vi "Initialize Measurement Actor Core.vi"(5 "Title Ref":refnum<vi>, 7 "Wvfm Graph Ref":refnum<vi>, 8 "error in (no error)":errorcluster, 11 "Measurement in":refnum<class "Function.lvclass">) -> (0 "error out":errorcluster, 1 "event out":refnum<user-event>, 2 "notifier out":refnum<notifier>, 3 "Measurement out":refnum<class "Function.lvclass">)   [LabVIEW 2016, in "Function Actor.lvlib" / "Function.lvclass"]
uses:
  <userlib>/Common Components/Function Actor/Function.lvclass
  C:/Program Files (x86)/National Instruments/LabVIEW 2016/vi.lib/ActorFramework/Actor/Actor.lvclass
  <userlib>/Common Components/Function Actor/Function.lvclass/Function.ctl
  <vilib>/ActorFramework/Actor/Actor.lvclass/Actor.ctl
  <vilib>/ActorFramework/Message Enqueuer/Message Enqueuer.lvclass/Message Enqueuer.ctl
  <vilib>/ActorFramework/Message Enqueuer/Enqueue.vi
  <vilib>/ActorFramework/Message Enqueuer/Init from Existing Queue.vi
  <userlib>/Common Components/Function Actor/Messages/Configure Msg/Configure Msg.lvclass
  C:/Program Files (x86)/National Instruments/LabVIEW 2016/vi.lib/ActorFramework/Message/Message.lvclass
  <vilib>/ActorFramework/Message Priority Queue/Priority Enqueue.vi
  <vilib>/ActorFramework/Message Enqueuer/Message Enqueuer.lvclass
  <vilib>/ActorFramework/Actor/Actor.lvclass
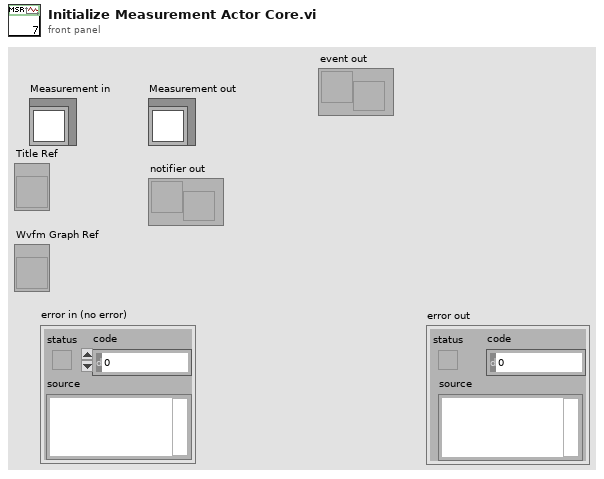
[diagram p1: front panel]
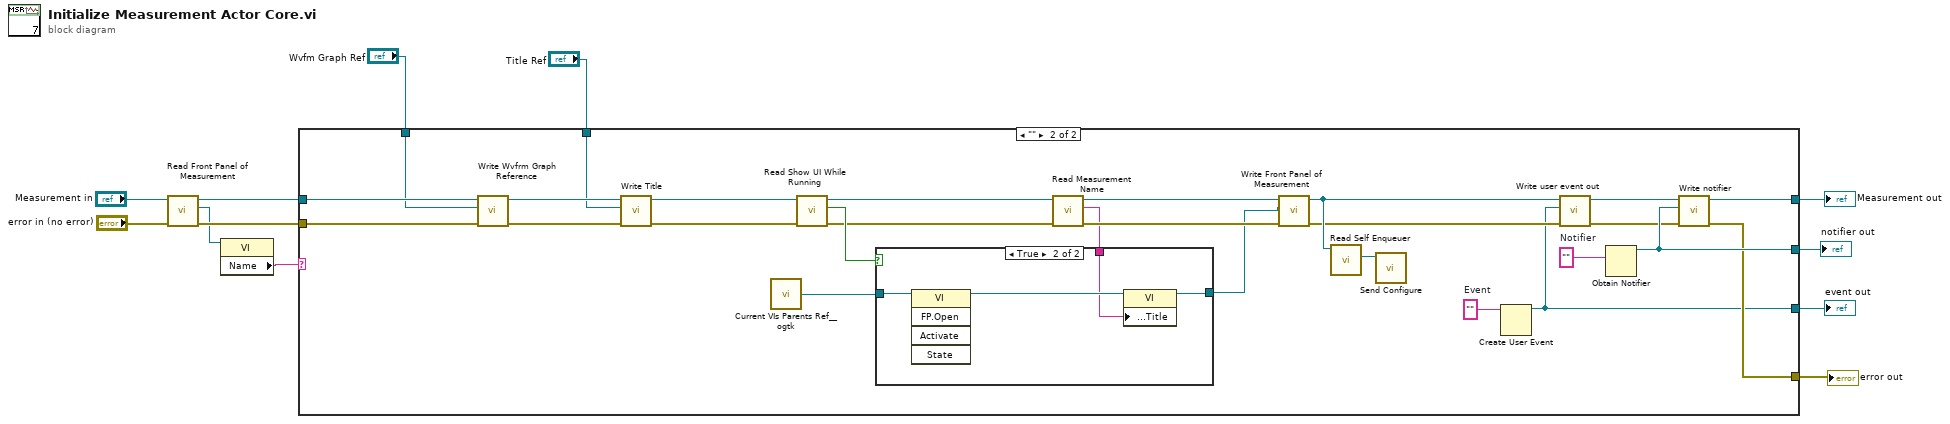
[diagram p0: block diagram]
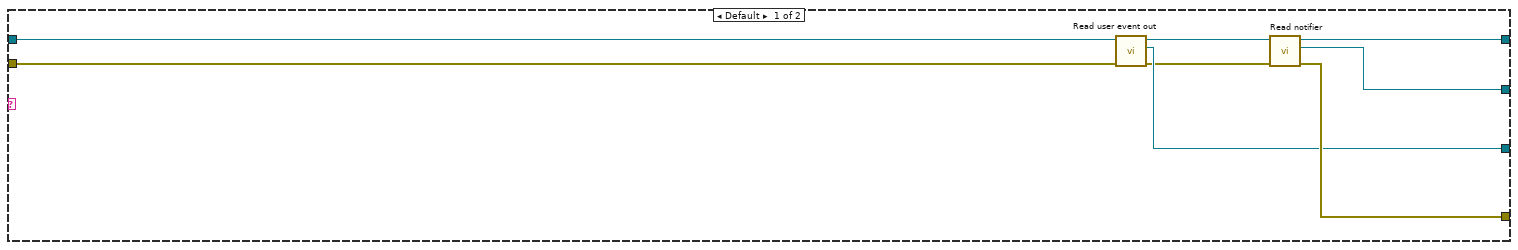
[diagram p2: hidden frame]
diagram:
  n1 = call <userlib>:"Read Front Panel of Measurement.vi"("error in (no error)"="error in (no error)", "Measurement in"="Measurement in") -> ("error out"=w9:errorcluster, "Front Panel of Measurement"=w8:refnum<vi>, "Measurement out"=w10:refnum<class "Function.lvclass">)  [unwired: 7 in]
  n2 = property class="VI"(reference=w8) -> ("Name"=w7:string)  [unwired: 1 in, 2 out]
  n3 = case shown="\"\"" w7 {
    tunnel: [w20 w46] -> w5
    tunnel: w10 -> [w17 w28]
    tunnel: w9 -> [w14 w27]
    tunnel: [w19 w45] -> w6
    tunnel: [w18 w44] -> w4
    tunnel: [w15 w29] -> w3
    tunnel: "Title Ref" -> [_ w22]
    tunnel: "Wvfm Graph Ref" -> [_ w21]
    frame Default {
      n4 = call <userlib>:"Read user event out.vi"("error in (no error)"=w14, "Measurement in"=w17) -> ("error out"=w13:errorcluster, "user event out"=w15:refnum<user-event>, "Measurement out"=w16:refnum<class "Function.lvclass">)  [unwired: 7 in]
      n5 = call <userlib>:"Read notifier.vi"("error in (no error)"=w13, "Measurement in"=w16) -> ("error out"=w18:errorcluster, "notifier"=w19:refnum<notifier>, "Measurement out"=w20:refnum<class "Function.lvclass">)  [unwired: 7 in]
    }
    frame "" {
      w34 = ""  # Event
      w47 = ""  # Notifier
      n6 = call <userlib>:"Write Wvfrm Graph Reference.vi"("error in (no error)"=w27, "General Measurement UI"=w21, "Measurement in"=w28) -> ("error out"=w26:errorcluster, "Measurement out"=w25:refnum<class "Function.lvclass">)  [unwired: 7 in]
      n7 = call <userlib>:"Write Title.vi"("error in (no error)"=w26, "Title"=w22, "Measurement in"=w25) -> ("error out"=w24:errorcluster, "Measurement out"=w23:refnum<class "Function.lvclass">)  [unwired: 7 in]
      n8 = call <userlib>:"Current VIs Parents Ref__ogtk.vi"() -> ("Calling VI's Reference"=w42:refnum<vi>)  [unwired: 2 in]
      n9 = call <userlib>:"Read Show UI While Running.vi"("error in (no error)"=w24, "Measurement in"=w23) -> ("error out"=w39:errorcluster, "Show UI While Running"=w41:bool, "Measurement out"=w40:refnum<class "Function.lvclass">)  [unwired: 7 in]
      n10 = call <userlib>:"Read Measurement Name.vi"("error in (no error)"=w39, "Measurement in"=w40) -> ("error out"=w38:errorcluster, "Measurement Name"=w35:string, "Measurement out"=w37:refnum<class "Function.lvclass">)  [unwired: 7 in]
      n11 = case shown="True" w41 {
        tunnel: w42 -> [w48 w52]
        tunnel: [w48 w50] -> w36
        tunnel: w35 -> [_ w49]
        frame False {
        }
        frame True {
          n12 = invoke class="VI" method="FP.Open"(reference=w52) -> (reference out=w51:refnum<vi>)  [unwired: 4 in, 4 out]
          n13 = property class="VI"(reference=w51, "Front Panel.Title"=w49) -> (reference out=w50:refnum<vi>)  [unwired: 1 in, 1 out]
        }
      }
      n14 = call <userlib>:"Write Front Panel of Measurement.vi"("error in (no error)"=w38, "Front Panel of Measurement"=w36, "Measurement in"=w37) -> ("error out"=w31:errorcluster, "Measurement out"=w33:refnum<class "Function.lvclass">)  [unwired: 7 in]
      n15 = call <vilib>:"Read Self Enqueuer.vi"("Actor"=w33) -> ("Self Enqueuer"=w43:refnum<class "Message Enqueuer.lvclass">)  [unwired: 10 in]
      n16 = call <userlib>:"Send Configure.vi"("Message Enqueuer in"=w43) -> ()  [unwired: 9 in, 2 out]
      n17 = Create User Event(user event datatype=w34) -> (user event=w29:refnum<user-event>)  [unwired: 1 in, 1 out]
      n18 = call <userlib>:"Write user event out.vi"("error in (no error)"=w31, "user event out"=w29, "Measurement in"=w33) -> ("error out"=w30:errorcluster, "Measurement out"=w32:refnum<class "Function.lvclass">)  [unwired: 7 in]
      n19 = Obtain Notifier(notification data type=w47) -> (notifier out=w45:refnum<notifier>)  [unwired: 3 in, 2 out]
      n20 = call <userlib>:"Write notifier.vi"("error in (no error)"=w30, "notifier"=w45, "Measurement in"=w32) -> ("error out"=w44:errorcluster, "Measurement out"=w46:refnum<class "Function.lvclass">)  [unwired: 7 in]
    }
  }
  "Measurement out" <- w5
  "error out" <- w4
  "notifier out" <- w6
  "event out" <- w3
